vi "HamburgerCB.vi"(4 "User Parameter":refnum<class "HamburgerMenu.lvclass">, 6 "Control":refnum<vi>, 7 "Event Common Data":cluster{"Source":T2, "Type":T3, "Time":u32} {"Source" items=["LabVIEW UI"=0, "ActiveX"=1, "User Event"=25]}) -> ()   [LabVIEW 2017, in "Hamburger Menu Library.lvlib" / "HamburgerMenu.lvclass"]
uses:
  HamburgerMenu/HamburgerMenu.lvclass
  <vilib>/event_ctls.llb/eventsource.ctl
  <vilib>/event_ctls.llb/lveventtype.ctl
  HamburgerMenu/HamburgerMenu.lvclass/HamburgerMenu.ctl
panel:
  in  "User Parameter old":T1
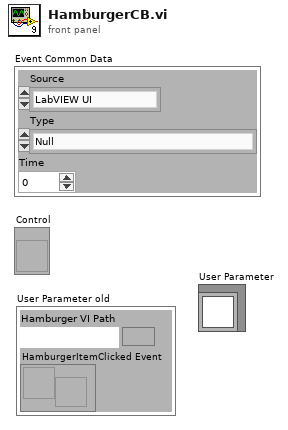
[diagram p1: front panel]
types:
  T1 = cluster{"Hamburger VI Path":path, "HamburgerItemClicked Event":refnum<user-event>}
  T2 = typedef "eventsource.ctl" = u32
  T3 = typedef "lveventtype.ctl" = enum32{"Null", "Timeout", "Annotation Menu Selection", "Annotation Menu Selection?", "App Instance Close", "App Instance Close?", "Autoscale Range Change", "Bookmark Info Change", "Cell Edit", "Cell Edit?", "Cursor Grab", "Cursor Grab?", "Cursor Menu Selection", "Cursor Menu Selection?", "Cursor Move", "Cursor Release", "Data Change", "Direction Change", "Display State Change", "Drag Ended", "Drag Enter", "Drag Leave", "Drag Over", "Drag Source Update", "Drag Starting", "Drag Starting?", "Drop", "Exec State Change", "Key Down", "Key Down?", "Key Repeat", "Key Repeat?", "Key Up", "Listbox Double Click", "Menu Activation?", "Menu Selection (App)", "Menu Selection? (App)", "Menu Selection (User)", "Mouse Down", "Mouse Down?", "Mouse Enter", "Mouse Leave", "Mouse Move", "Mouse Up", "Mouse Wheel", "NI Security User Change (App)", "Pane Size", "Panel Close", "Panel Close?", "Panel Resize", "Plot Attribute Change", "Scale Range Change", "Shortcut Menu Activation?", "Shortcut Menu Selection (App)", "Shortcut Menu Selection? (App)", "Shortcut Menu Selection (User)", "Tree Double Click", "Tree Drag", "Tree Drag?", "Tree Drop", "Tree Drop?", "Tree Item Close", "Tree Item Close?", "Tree Item Open", "Tree Item Open?", "User Event", "Value Change"}
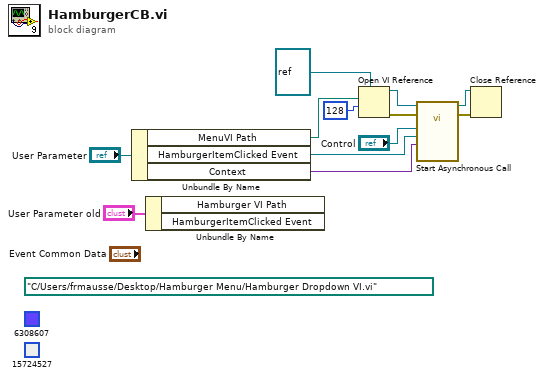
[diagram p0: block diagram]
diagram:
  (unwired) u32 15724527
  (unwired) u32 6308607
  (unwired) path "C:/Users/frmausse/Desktop/Hamburger Menu/Hamburger Dropdown VI.vi" ("vi path")
  n1 = Unbundle By Name("User Parameter") -> ("MenuVI Path"=w3:path, "HamburgerItemClicked Event"=w2:refnum<user-event>, "Context"=w1:variant)
  n2 = Unbundle By Name("User Parameter old") -> ()  [unwired: 2 out]
  n3 = Open VI Reference(type specifier VI Refnum (for type only)=refnum<vi> refnum, vi path=w3, options=128) -> (vi reference=w10:refnum<vi>, error out=w9:errorcluster)  [unwired: 3 in]
  n4 = call-by-ref "Start Asynchronous Call"(reference=w10, error in=w9, "Context"=w1, "HamburgerItemClicked Event"=w2, "HamburgerCtl Ref"="Control") -> (reference out=w7:refnum<vi>, error out=w8:errorcluster)  [unwired: 9 in]
  n5 = Close Reference(reference=w7, error in (no error)=w8) -> ()  [unwired: 1 out]
